vi "_intersectReactivity.vi"(10 "反应性":dbl[](array[numeric]), 11 "通量":dbl[](array[numeric])) -> (2 "通量+反应性":dbl[](array[numeric]))   [LabVIEW 2020]
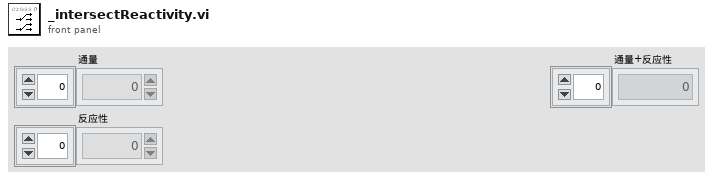
[diagram p1: front panel]
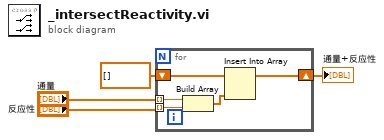
[diagram p0: block diagram]
diagram:
  n1 = for {
    tunnel: "通量" -> [w7] mode=indexing
    tunnel: "反应性" -> [w6] mode=indexing
    shift-right: [w8] -> w3
    shift-left: dbl[] [] -> [w9]
    n2 = Build Array(w7, w6) -> (w5:dbl[])
    n3 = Insert Into Array(array=w9, new element=w5) -> (w8:dbl[])  [unwired: 1 in]
  }
  "通量+反应性" <- w3
